vi "FGV_MBmaster(RTU).vi"(4 "flow control (None)":u16(ring) items=["None", "XON/XOFF", "RTS/CTS", "XON/XOFF & RTS/CTS", "DTR/DSR", "XON/XOFF & DTR/DSR"], 6 "parity (Even)":u16(ring)=2 items=["None", "Odd", "Even"], 7 "FV_MBmaster(RTU)":T1, 8 "error in (no error)":errorcluster, 9 "holding register values":u16[](array[numeric]), 10 "baud rate (9600)":u32=9600, 11 "VISA resource name":refnum<visa-resource-name>) -> (0 "error out":errorcluster, 2 "register values":u16[](array[numeric]))   [LabVIEW 2017]
uses:
  Controls/FV_MBmuster(RTU).ctl
  <vilib>/Modbus/master/Modbus Master.lvclass
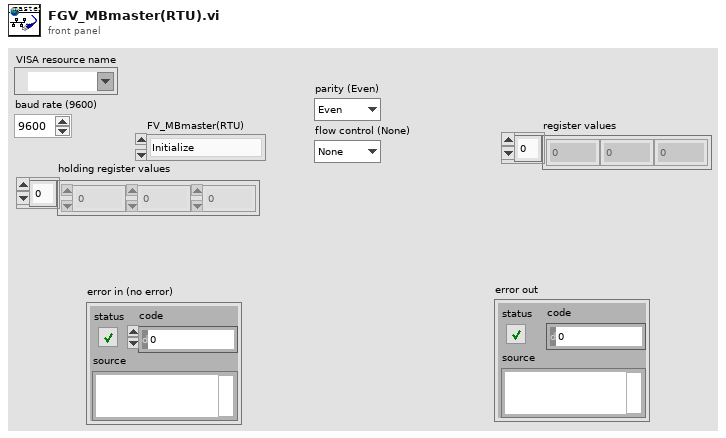
[diagram p1: front panel]
types:
  T1 = typedef "FV_MBmuster(RTU).ctl" = enum16{"Initialize", "Create Master", "Write Register", "Read Register", "Close Master"}
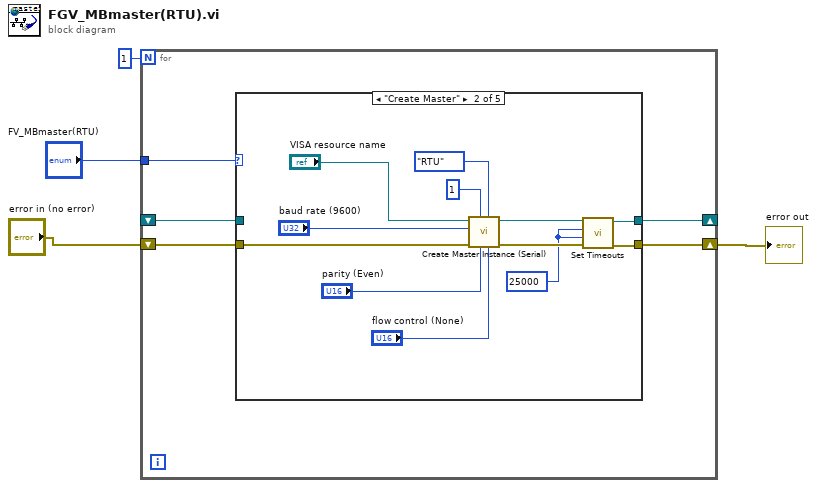
[diagram p0: block diagram]
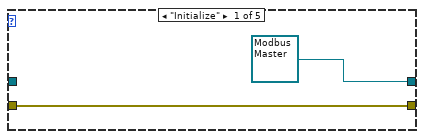
[diagram p2: hidden frame]
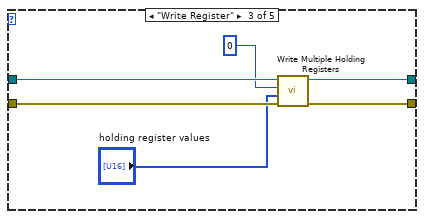
[diagram p3: hidden frame]
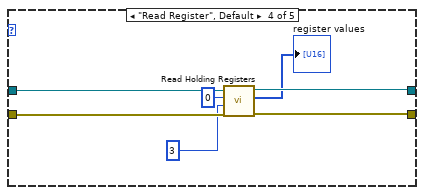
[diagram p4: hidden frame]
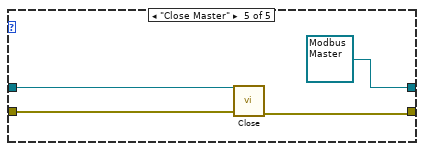
[diagram p5: hidden frame]
diagram:
  n1 = for {
    N: 1 -> [_]
    tunnel: "FV_MBmaster(RTU)" -> [w9]
    shift-right: [w8] -> w2
    shift-left: "error in (no error)" -> [w7]
    shift-right: [w6] -> _
    shift-left: _ -> [w5]
    n2 = case shown="\"Create Master\"" w9 {
      tunnel: [w11 w14 w28 w34 w39] -> w8
      tunnel: w7 -> [w11 w20 w29 w35 w40]
      tunnel: [refnum<class "Modbus Master.lvclass"> refnum ("Modbus master out") w13 w27 w33 refnum<class "Modbus Master.lvclass"> refnum ("Modbus master out")] -> w6
      tunnel: w5 -> [_ _ w26 w36 w38]
      frame "Initialize" {
      }
      frame "Create Master" {
        w12 = 25000 ("write operation timeout (ms)")
        n3 = call <vilib>:"Create Master Instance (Serial).vi"("flow control (None)"="flow control (None)", "serial type"=enum16{"RTU", "ASCII"}."RTU", "parity (Even)"="parity (Even)", "unit ID"=u8 1, "error in (no error)"=w20, "baud rate (9600)"="baud rate (9600)", "VISA resource name"="VISA resource name") -> ("error out"=w15:errorcluster, "serial master instance"=w16:refnum<class "Modbus Master.lvclass">)  [unwired: 3 in]
        n4 = call <vilib>:"Set Timeouts.vi"("error in (no error)"=w15, "write operation timeout (ms)"=w12, "read operation timeout (ms)"=w12, "Modbus master in"=w16) -> ("error out"=w14:errorcluster, "Modbus master out"=w13:refnum<class "Modbus Master.lvclass">)  [unwired: 6 in]
      }
      frame "Write Register" {
        n5 = call-dynamic "Write Multiple Holding Registers.vi"("error in (no error)"=w29, "holding register values"="holding register values", "starting address"=u16 0, "Modbus master in"=w26) -> ("error out"=w28:errorcluster, "Modbus master out"=w27:refnum<class "Modbus Master.lvclass">)  [unwired: 6 in]
      }
      frame "Read Register", Default {
        n6 = call-dynamic "Read Holding Registers.vi"("error in (no error)"=w35, "number of holding registers"=u16 3, "starting address"=u16 0, "Modbus master in"=w36) -> ("error out"=w34:errorcluster, "register values"=→"register values":u16[], "Modbus master out"=w33:refnum<class "Modbus Master.lvclass">)  [unwired: 5 in]
      }
      frame "Close Master" {
        n7 = call-dynamic "Close.vi"("error in (no error)"=w40, "Modbus master in"=w38) -> ("error out"=w39:errorcluster)  [unwired: 9 in]
      }
    }
  }
  "error out" <- w2
